vi "LV_exo1v3_cleaned_up.vi"() -> ()   [LabVIEW 2023]
panel:
  in  "marker size":i32
  in  "marker type":string
  out "Colours":u32[](array[colorbox])
  out "output matlab":string
  out "error out 2":errorcluster
  out "standard error":string
  out "standard output":string
  out "Scanned Image":picture
  in  "Path":path
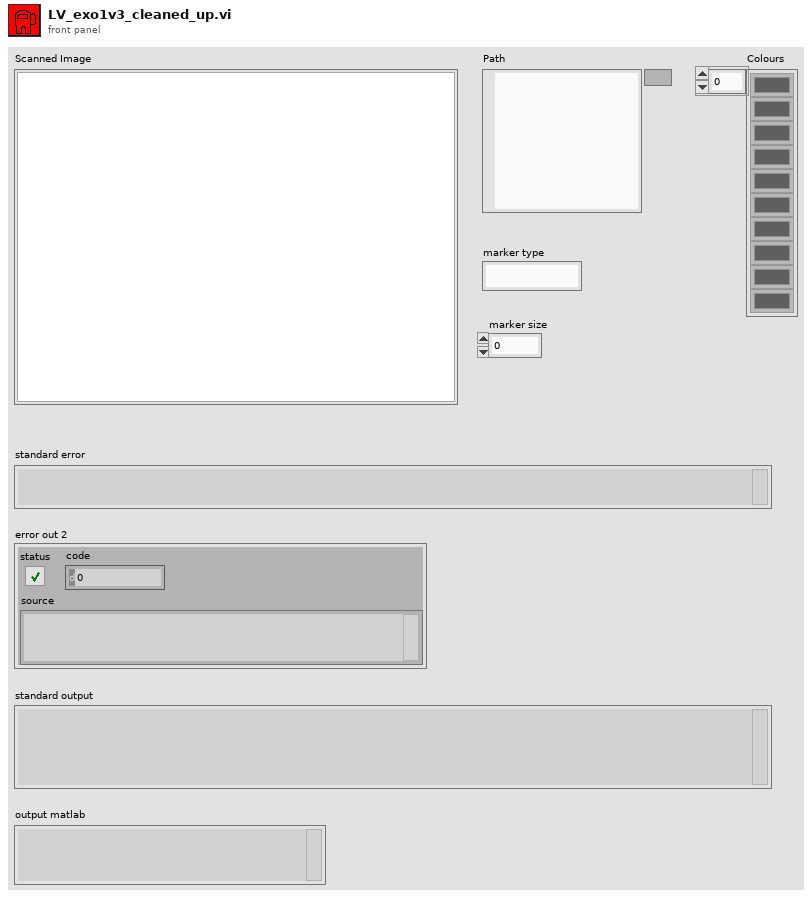
[diagram p1: front panel]
types:
  T1 = enum16{"big-endian, network order", "native, host order", "little-endian"}
  T2 = typedef "imagedata.ctl" = cluster{"image type":i32, "image depth":i32, "image":u8[], "mask":u8[], "colors":u32[], "Rectangle":cluster{"left":i16, "top":i16, "right":i16, "bottom":i16}}
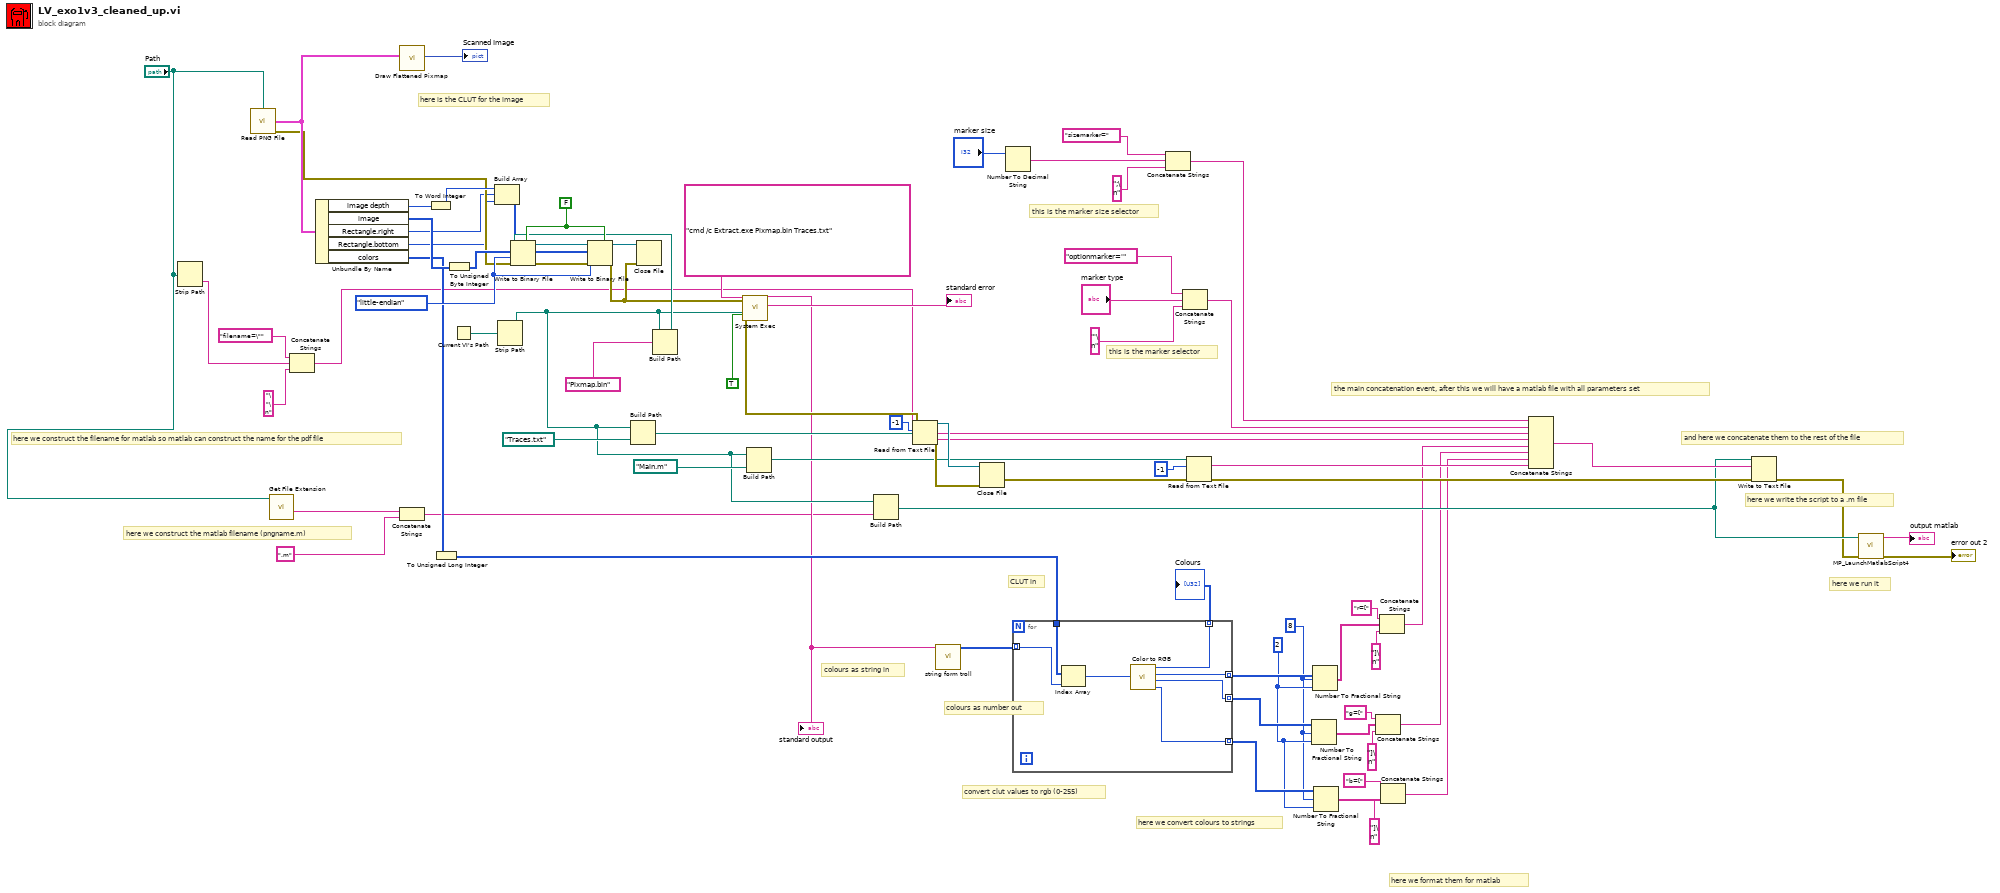
[diagram p0: block diagram]
diagram:
  w27 = i16 2 ("precision (6)")
  w26 = i16 8 ("width (-)")
  w71 = T1."little-endian" ("byte order (0:big-endian, network order)")
  w77 = FALSE
  # "this is the marker size selector"
  # "here we construct the matlab filename (pngname.m)"
  # "colours as number out"
  # "colours as string in"
  # "CLUT in"
  # "here is the CLUT for the image"
  # "convert clut values to rgb (0-255)"
  # "here we run it"
  # "here we write the script to a .m file"
  # "here we construct the filename for matlab so matlab can construct the name for the pdf file"
  # "the main concatenation event, after this we will have a matlab file with all parameters set"
  # "this is the marker selector"
  # "and here we concatenate them to the rest of the file"
  # "here we format them for matlab"
  # "here we convert colours to strings"
  n1 = Strip Path(path="Path") -> (name=w43:string)  [unwired: 1 out]
  n2 = call <vilib>:"Read PNG File.vi"("path to PNG file"="Path") -> ("error out"=w56:errorcluster, "image data"=w75:T2)  [unwired: 8 in, 1 out]
  n3 = call <vilib>:"Get File Extension.vi"("file"="Path") -> ("filename without extension"=w8:string)  [unwired: 6 in, 4 out]
  n4 = Concatenate Strings("filename=\"" ("string"), w43, "\"\n" ("string")) -> (w34:string)
  n5 = Unbundle By Name(w75) -> ("image depth"=w78:i32, "image"=w40:u8[], "Rectangle.right"=w11:i16, "Rectangle.bottom"=w10:i16, "colors"=w39:u32[])
  n6 = call <vilib>:"Draw Flattened Pixmap.vi"("image data"=w75) -> ("new picture"=→"Scanned Image":picture)  [unwired: 8 in]
  n7 = Concatenate Strings(w8, ".m" ("string")) -> (w6:string)
  n8 = To Word Integer(number=w78) -> (16bit integer=w79:i16)
  n9 = To Unsigned Long Integer(number=w39) -> (unsigned 32bit integer=w38:u32[])
  n10 = To Unsigned Byte Integer(number=w40) -> (unsigned 8bit integer=w64:u8[])
  n11 = Current VI's Path() -> (path=w69:path)
  n12 = Build Array(w79, w11, w10) -> (w65:i16[])
  n13 = Strip Path(path=w69) -> (stripped path=w48:path)  [unwired: 1 out]
  n14 = Build Path(base path=w48, name or relative path=path "Traces.txt") -> (appended path=w61:path)
  n15 = Build Path(base path=w48, name or relative path="Pixmap.bin" ("String")) -> (appended path=w70:path)
  n16 = Write to Binary File(file (use dialog)=w70, data=w65, error in=w56, 5:w77, 9:w71) -> (refnum out=w63:refnum<file>, error out=w76:errorcluster)  [unwired: 1 in, 1 out]
  n17 = Write to Binary File(file (use dialog)=w63, data=w64, error in=w76, 5:w77, 9:w71) -> (refnum out=w66:refnum<file>, error out=w67:errorcluster)  [unwired: 1 in, 1 out]
  n18 = Close File(refnum=w66, error in=w67) -> ()  [unwired: 2 out]
  n19 = call <vilib>:"System Exec.vi"("run minimized? (F)"=TRUE, "error in (no error)"=w67, "working directory"=w48, "command line"="cmd /c Extract.exe Pixmap.bin Traces.txt") -> ("error out"=w60:errorcluster, "standard error"=→"standard error":string, "standard output"=w37:string)  [unwired: 4 in, 1 out]
  "standard output" <- w37
  n20 = Build Path(base path=w48, name or relative path=path "Main.m") -> (appended path=w53:path)
  n21 = Build Path(base path=w48, name or relative path=w6) -> (appended path=w47:path)
  n22 = Read from Text File(file (use dialog)=w61, count=-1, error in=w60) -> (refnum out=w58:refnum<file>, text=w55:string, error out=w57:errorcluster)  [unwired: 1 in, 1 out]
  n23 = call "string form troll.vi"("String"=w37) -> ("Array"=w36:u32[])  [unwired: 10 in]
  n24 = Close File(refnum=w58, error in=w57) -> (error out=w52:errorcluster)  [unwired: 1 out]
  n25 = Number To Decimal String(number="marker size") -> (decimal integer string=w3:string)  [unwired: 1 in]
  n26 = for {
    tunnel: w36 -> [w87] mode=indexing
    tunnel: w38 -> [w86]
    tunnel: [w85] -> w32 mode=indexing
    tunnel: [w84] -> w33 mode=indexing
    tunnel: [w83] -> w31 mode=indexing
    tunnel: [w81] -> w35 mode=indexing
    n27 = Index Array(array=w86, index=w87) -> (element=w82:u32)
    n28 = call <vilib>:"Color to RGB.vi"("Color"=w82) -> ("Resolved Color"=w81:u32, "R"=w85:u8, "G"=w84:u8, "B"=w83:u8)
  }
  "Colours" <- w35
  n29 = Concatenate Strings("sizemarker=" ("string"), w3, ";\n" ("string")) -> (w1:string)
  n30 = Concatenate Strings("optionmarker='" ("string"), "marker type", "'\n" ("string")) -> (w15:string)
  n31 = Read from Text File(file (use dialog)=w53, count=-1, error in=w52) -> (text=w19:string, error out=w49:errorcluster)  [unwired: 1 in, 2 out]
  n32 = Number To Fractional String(number=w33, width (-)=w26, precision (6)=w27) -> (F-format string=w21:string[])  [unwired: 1 in]
  n33 = Number To Fractional String(number=w32, width (-)=w26, precision (6)=w27) -> (F-format string=w30:string[])  [unwired: 1 in]
  n34 = Number To Fractional String(number=w31, width (-)=w26, precision (6)=w27) -> (F-format string=w20:string[])  [unwired: 1 in]
  n35 = Concatenate Strings("g=[" ("string"), w21, "]\n" ("string")) -> (w17:string)
  n36 = Concatenate Strings("r=[" ("string"), w30, "]\n" ("string")) -> (w18:string)
  n37 = Concatenate Strings("b=[" ("string"), w20, "]\n" ("string")) -> (w16:string)
  n38 = Concatenate Strings(w1, w15, w55, w34, w18, w17, w16, w19) -> (w50:string)
  n39 = Write to Text File(file (use dialog)=w47, text=w50, error in=w49) -> (error out=w45:errorcluster)  [unwired: 1 in, 2 out]
  n40 = call "MP_LaunchMatlabScript4.vi"("error in (no error)"=w45, "matlab script path"=w47) -> ("error out"=→"error out 2":errorcluster, "standard output"=→"output matlab":string)  [unwired: 4 in, 4 out]
